vi "Running HP34401 Average.vi"(2 "Point #":i32, 3 "Instrument Address":refnum<visa-resource-name>) -> (0 "Stop":bool, 1 "?":dbl[](array[numeric]) format="%.4e")   [LabVIEW 2021]
doc: "This VI takes a running difference of 3 measurements of a HP34401 DMM. It assumes that the current has been reversed for the middle measurements. The value returned is the average of the 1st and 3rd measurements minus the 2nd measurement over 2.\nScott Hannahs, NHMFL - FSU, April 1995"
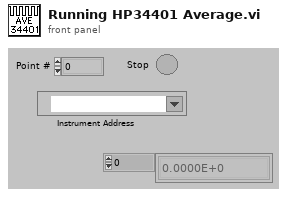
[diagram p1: front panel]
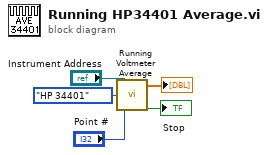
[diagram p0: block diagram]
diagram:
  n1 = call "Running Voltmeter Average.vi"("Point #"="Point #", "Type"=enum16{"DMM", "HP 34401", "Keithley 2001"}."HP 34401", "Instrument Address"="Instrument Address") -> ("Stop"=→"Stop":bool, 1:→"?":dbl[])
